vi "Sea-Level Download SeaIo32.dll.vi"(1 "Driver Path":string) -> (0 "New Driver Path":string)   [LabVIEW 2011]
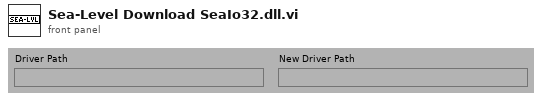
[diagram p1: front panel]
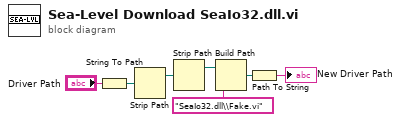
[diagram p0: block diagram]
diagram:
  n1 = String To Path(string="Driver Path") -> (path=w6:path)
  n2 = Strip Path(path=w6) -> (stripped path=w5:path)  [unwired: 1 out]
  n3 = Strip Path(path=w5) -> (stripped path=w4:path)  [unwired: 1 out]
  n4 = Build Path(base path=w4, name or relative path="SeaIo32.dll\\Fake.vi") -> (appended path=w2:path)
  n5 = Path To String(path=w2) -> (string=→"New Driver Path":string)
